vi "Multi (Selector).vi"(8 "error in (no error)":errorcluster, 9 "Constant":dbl=1.0, 10 "Aux Data Sources":T1) -> (0 "error out":errorcluster, 3 "Multi out":refnum<class "Multi.lvclass">)   [LabVIEW 2009, in "Multi.lvclass"]
uses:
  Multi.lvclass
  Average/Average.lvclass
  Difference/Difference.lvclass
  Plus/Plus.lvclass
  Multiply/Multiply.lvclass
  Polarization/Polarization.lvclass
  Normalize/Normalize.lvclass
  Norm/Norm.lvclass
  Aux Data Source/Aux Data Source.lvclass
  Phase/Phase.lvclass
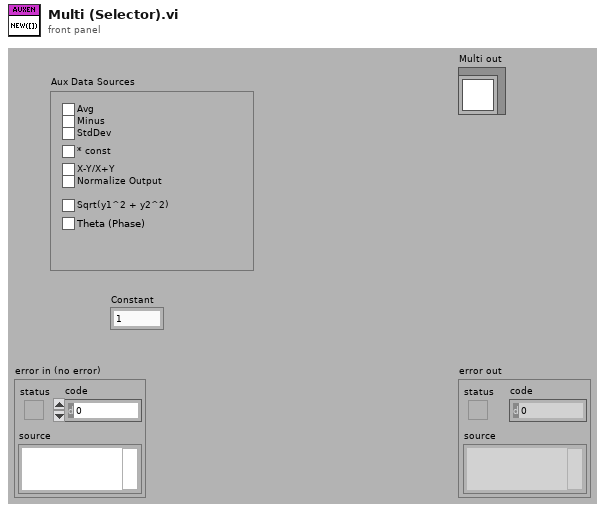
[diagram p1: front panel]
types:
  T1 = cluster{"Avg":bool, "Minus":bool, "StdDev":bool, "* const":bool, "X-Y/X+Y":bool, "Normalize Output":bool, "Sqrt(y1^2 + y2^2)":bool, "Theta (Phase)":bool}
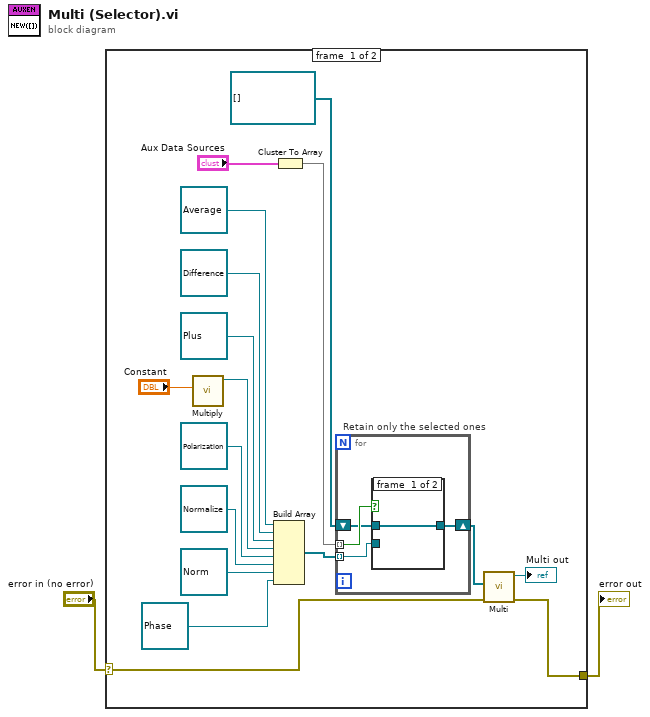
[diagram p0: block diagram]
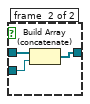
[diagram p2: hidden frame]
diagram:
  n1 = case shown="No Error" "error in (no error)" {
    selector: "error in (no error)" -> [w9 w28]
    tunnel: [w8 w28] -> w1
    frame #0 {
      n2 = call "Multiply.vi"("Constant"="Constant") -> ("Multiply out"=w15:refnum<class "Multiply.lvclass">)  [unwired: 9 in, 1 out]
      n3 = Build Array(refnum<class "Average.lvclass"> refnum ("Average.lvclass"), refnum<class "Difference.lvclass"> refnum ("Difference.lvclass"), refnum<class "Plus.lvclass"> refnum ("Plus.lvclass"), w15, refnum<class "Polarization.lvclass"> refnum ("Polarization.lvclass"), refnum<class "Normalize.lvclass"> refnum ("Normalize.lvclass"), refnum<class "Norm.lvclass"> refnum ("Norm.lvclass"), refnum<class "Phase.lvclass"> refnum ("Phase.lvclass")) -> (w11:refnum<class>[])
      n4 = Cluster To Array(cluster="Aux Data Sources") -> (array=w12:bool[])
      n5 = for "Retain only the selected ones" {
        tunnel: w12 -> [w22] mode=indexing
        tunnel: w11 -> [w23] mode=indexing
        shift-right: [w20] -> w10
        shift-left: refnum<class "Aux Data Source.lvclass">[] [] -> [w21]
        n6 = case shown="True" w22 {
          tunnel: w23 -> [_ w26]
          tunnel: [w24 w27] -> w20
          tunnel: w21 -> [w24 w25]
          frame #0 {
          }
          frame #1 {
            n7 = Build Array (concatenate)(w25, w26) -> (w27:refnum<class>[])
          }
        }
      }
      n8 = call "Multi.vi"("error in (no error)"=w9, "Data Sources"=w10) -> ("error out"=w8:errorcluster, "Multi out"=→"Multi out":refnum<class "Multi.lvclass">)  [unwired: 8 in]
    }
    frame #1 {
    }
  }
  "error out" <- w1
